vi "Get Object ACL.vi"(4 "Region":T1, 6 "Version ID":string, 8 "error in (no error)":errorcluster, 9 "Bucket":string, 10 "Object Path":string) -> (0 "error out":errorcluster, 3 "AccessControlPolicy":T2)   [LabVIEW 2015, in "LV Interface for Amazon S3.lvlib"]
doc: "This operation <B>returns the access control list (ACL)</B> of an object. To use this operation, <B>you must have READ_ACP access</B> to the object."
uses:
  LV Interface for Amazon S3.lvlib
  Typedefs/AMZ_S3_API_AccessControlPolicy.ctl
  Typedefs/AMZ_S3_API_Owner.ctl
  Typedefs/AMZ_S3_API_Bucket ACL Permission.ctl
  Typedefs/AMZ_S3_LocationConstraint.ctl
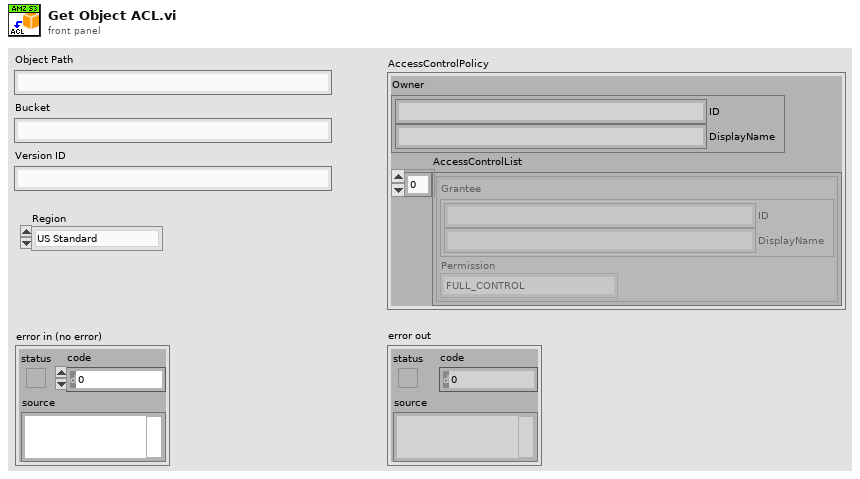
[diagram p1: front panel]
types:
  T1 = typedef "LV Interface for Amazon S3.lvlib/AMZ_S3_LocationConstraint.ctl" = enum16{"US Standard", "us-east-2", "us-west-1", "us-west-2", "ap-northeast-1", "ap-northeast-2", "ap-southeast-1", "ap-southeast-2", "ca-central-1", "eu-central-1", "eu-west-1", "eu-west-2", "sa-east-1"}
  T2 = typedef "LV Interface for Amazon S3.lvlib/AMZ_S3_API_AccessControlPolicy.ctl" = cluster{"Owner":T3, "AccessControlList":cluster{"Grantee":T3, "Permission":T4}[]}
  T3 = typedef "LV Interface for Amazon S3.lvlib/AMZ_S3_API_Owner.ctl" = cluster{"ID":string, "DisplayName":string}
  T4 = typedef "LV Interface for Amazon S3.lvlib/AMZ_S3_API_Bucket ACL Permission.ctl" = enum16{"FULL_CONTROL", "WRITE", "WRITE_ACP", "READ", "READ_ACP"}
  T5 = cluster{"format string":string, "Version ID":string}
  T6 = cluster{"format string":string, "Version ID":string}[]
  T7 = typedef "LV Interface for Amazon S3.lvlib/AMZ_S3_Call Results.ctl" = enum16{"Success", "UndefinedError", "AccessDenied", "AccountProblem", "AmbiguousGrantByEmailAddress", "BadDigest", "BucketAlreadyExists", "BucketAlreadyOwnedByYou", "BucketNotEmpty", "CredentialsNotSupported", "CrossLocationLoggingProhibited", "EntityTooSmall", "EntityTooLarge", "ExpiredToken", "IllegalVersioningConfigurationException", "IncompleteBody", "IncorrectNumberOfFilesInPostRequest", "InlineDataTooLarge", "InternalError", "InvalidAccessKeyId", "InvalidAddressingHeader", "InvalidArgument", "InvalidBucketName", "InvalidDigest", "InvalidLocationConstraint", "InvalidPart", "InvalidPartOrder", "InvalidPayer", "InvalidPolicyDocument", "InvalidRange", "InvalidSecurity", "InvalidSOAPRequest", "InvalidStorageClass", "InvalidTargetBucketForLogging", "InvalidToken", "InvalidURI", "KeyTooLong", "MalformedACLError", "MalformedPOSTRequest", "MalformedXML", "MaxMessageLengthExceeded", "MaxPostPreDataLengthExceededError", "MetadataTooLarge", "MethodNotAllowed", "MissingAttachment", "MissingContentLength", "MissingRequestBodyError", "MissingSecurityElement", "MissingSecurityHeader", "NoLoggingStatusForKey", "NoSuchBucket", "NoSuchKey", "NoSuchUpload", "NoSuchVersion", "NotImplemented", "NotSignedUp", "OperationAborted", "PermanentRedirect", "PreconditionFailed", "Redirect", "RequestIsNotMultiPartContent", "RequestTimeout", "RequestTimeTooSkewed", "RequestTorrentOfBucketError", "SignatureDoesNotMatch", "SlowDown", "TemporaryRedirect", "TokenRefreshRequired", "TooManyBuckets", "UnexpectedContent", "UnresolvableGrantByEmailAddress", "UserKeyMustBeSpecified", "LabVIEWError"}
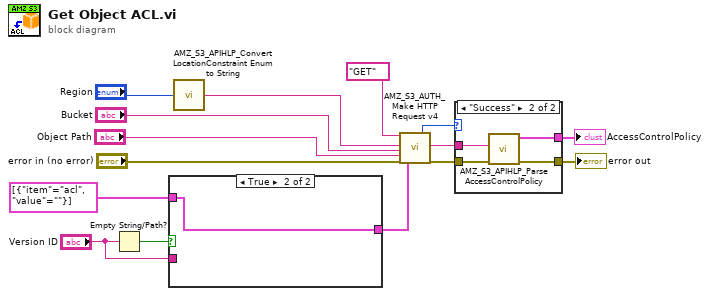
[diagram p0: block diagram]
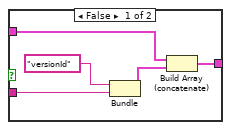
[diagram p2: hidden frame]
diagram:
  n1 = Empty String/Path?(string/path="Version ID") -> (empty?=w12:bool)
  n2 = case shown="True" w12 {
    tunnel: cluster{"item":string, "value":string}[] [{"item"="acl", "value"=""}] ("request parameters") -> [w19 w21]
    tunnel: "Version ID" -> [w17 _]
    tunnel: [w16 w21] -> w3
    frame False {
      n3 = Bundle("format string"="versionId", "Version ID"=w17) -> (w18:T5)  [unwired: 1 in]
      n4 = Build Array (concatenate)(w19, w18) -> (w16:T6)
    }
    frame True {
    }
  }
  n5 = call "AMZ_S3_APIHLP_Convert LocationConstraint Enum to String.vi"("Location"="Region") -> ("Location String"=w1:string)  [unwired: 4 in]
  n6 = call "AMZ_S3_AUTH_Make HTTP Request v4.vi"("HTTP-Verb"="GET", "Region"=w1, "Bucket"="Bucket", "Object Key"="Object Path", "error in"="error in (no error)", "request parameters"=w3) -> ("Call Result"=w8:T7, "response body"=w9:string, "error out"=w10:errorcluster)  [unwired: 10 in, 1 out]
  n7 = case shown="\"Success\"" w8 {
    tunnel: w10 -> [w22 w26]
    tunnel: w9 -> [_ w25]
    tunnel: [w22 w24] -> w14
    tunnel: [_ w23] -> w15
    frame Default {
    }
    frame "Success" {
      n8 = call "AMZ_S3_APIHLP_Parse AccessControlPolicy.vi"("error in (no error)"=w26, "Response body"=w25) -> ("error out"=w24:errorcluster, "AccessControlPolicy"=w23:T2)  [unwired: 8 in]
    }
  }
  "AccessControlPolicy" <- w15
  "error out" <- w14
